vi "Handle Connection Error.vi"(8 "error in (no error)":errorcluster) -> (0 "error in (no error) 2":errorcluster)   [LabVIEW 2025, in "Power Supply.lvlib"]
uses:
  Power Supply.lvlib
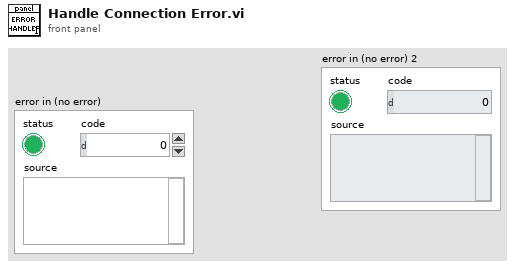
[diagram p1: front panel]
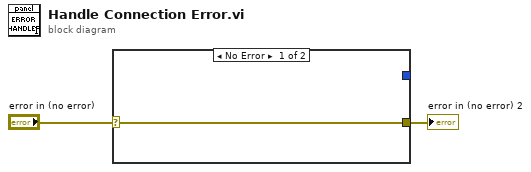
[diagram p0: block diagram]
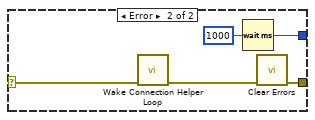
[diagram p2: hidden frame]
diagram:
  n1 = case shown="No Error" "error in (no error)" {
    selector: "error in (no error)" -> [w3 w6]
    tunnel: [w3 w7] -> w2
    tunnel: [_ w5] -> _
    frame No Error {
    }
    frame Error {
      n2 = call "Wake Connection Helper Loop.vi"("error in"=w6) -> ("error out"=w8:errorcluster)  [unwired: 10 in]
      n3 = Wait (ms)(milliseconds to wait=u32 1000) -> (millisecond timer value=w5:u32)
      n4 = call <vilib>:"Clear Errors.vi"("error in (no error)"=w8) -> ("error out"=w7:errorcluster)  [unwired: 5 in, 1 out]
    }
  }
  "error in (no error) 2" <- w2
